vi "Sub_Close.vi"(0 "DeviceHandle":u32) -> ()   [LabVIEW 2013]
uses:
  documentation/SDK/x64_lib/Mightex_LEDDriver_SDK.dll
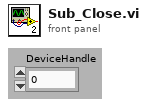
[diagram p1: front panel]
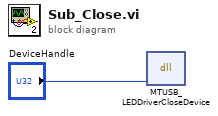
[diagram p0: block diagram]
diagram:
  n1 = dll-call lib="C:/Users/ignacio/Desktop/Patrick's File Reader Function/led_control/documentation/SDK/x64_lib/Mightex_LEDDriver_SDK.dll" fn="MTUSB_LEDDriverCloseDevice"("arg1"="DeviceHandle") -> ()  [unwired: 5 in, 2 out]
